vi "init.vi"(0 "Camera in":refnum<class "Camera.lvclass">, 1 "interface":u8(ring)=255 items=["FireWire"=1, "GenICam"=3, "GigE"=5, "USB"=6, "CameraLinkME4"=7, "USB3"=8, "CLHS"=11, "All"=255], 3 "error in (no error)":errorcluster) -> (7 "Camera out":refnum<class "Camera.lvclass">, 10 "error out":errorcluster)   [LabVIEW 2019, in "Camera.lvclass"]
doc: "This function is similar to init.vi but with the additional option to select the interface where\ncameras should be searched for. The default is All Interfaces. In contrast to init.vi, this function\nuses the pco.sdk function PCO_OpenCameraEx.vi to search the interfaces individually.\n\nYou should use this function instead of init.vi when:\n - You want to search for cameras at a specific interface.\n - You want to create multiple Camera objects in an application where the cameras are partially connected during operation."
uses:
  Camera.lvclass
  pco.sdk/Structures/Structures.lvlib
  pco.sdk/CameraAccess/CameraAccess.lvlib
  pco.sdk/CameraDescription/CameraDescription.lvlib
  pco.sdk/GeneralCameraStatus/GeneralCameraStatus.lvlib
  pco.convert/Convert.lvlib
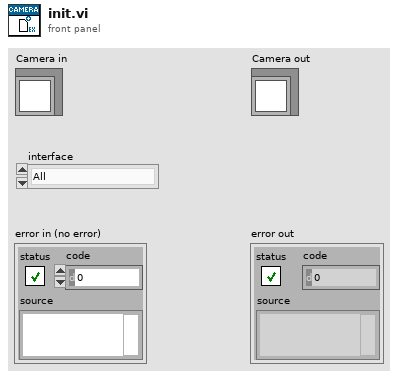
[diagram p1: front panel]
types:
  T1 = cluster{"wCamType":u16, "wCamSubType":u16, "dwSerialNumber":u32, "dwHWVersion":u32, "dwFWVersion":u32, "InterfaceType":u16, "PCO_FW_Vers":cluster{"wDeviceNum":u16, "PCO_SC2_Firmware_DESC":cluster{"szName":string, "bMinorRev":u8, "bMajorRev":u8, "wVariant":u16}[]}, "PCO_HW_Vers":cluster{"wBoardNum":u16, "PCO_SC2_Hardware_DESC":cluster{"szName":string, "wBatchNo":u16, "wRevision":u16, "wVariant":u16}[]}}
  T2 = cluster{"wSensorTypeDESC":u16, "wSensorSubTypeDESC":u16, "wMaxHorzResStdDESC":u16, "wMaxVertResStdDESC":u16, "wMaxHorzResExtDESC":u16, "wMaxVertResExtDESC":u16, "wDynResDESC":u16, "wMaxBinHorzDESC":u16, "wBinHorzSteppingDESC":u16, "wMaxBinVertDESC":u16, "wBinVertSteppingDESC":u16, "wRoiHorStepsDESC":u16, "wRoiVertStepsDESC":u16, "wNumADCsDESC":u16, "wMinSizeHorzDESC":u16, "dwPixelRateDESC":u32[], "wConvFactDESC":u16[], "sCoolingSetpoints":i16[], "wSoftRoiHorStepsDESC":u16, "wSoftRoiVertStepsDESC":u16, "wIRDESC":u16, "wMinSizeVertDESC":u16, "dwMinDelayDESC":u32, "dwMaxDelayDESC":u32, "dwMinDelayStepDESC":u32, "dwMinExposureDESC":u32, "dwMaxExposureDESC":u32, "dwMinExposureStepDESC":u32, "dwMinDelayIRDESC":u32, "dwMaxDelayIRDESC":u32, "dwMinExposureIRDESC":u32, "dwMaxExposureIRDESC":u32, "wTimeTableDESC":u16, "wDoubleImageDESC":u16, "sMinCoolSetDESC":i16, "sMaxCoolSetDESC":i16, "sDefaultCoolSetDESC":i16, "wPowerDownModeDESC":u16, "wOffsetRegulationDESC":u16, "wColorPatternDESC":u16, "wPatternTypeDESC":u16, "wNumCoolingSetpoints":u16, "dwGeneralCapsDESC1":u32, "dwGeneralCapsDESC2":u32, "dwExtSyncFrequency":u32[], "dwGeneralCapsDESC3":u32, "dwGeneralCapsDESC4":u32}
  T3 = cluster{"sharpen":bool, "adaptive_sharpen":bool, "flip_vertical":bool, "auto_minmax":bool, "min_limit":u16, "max_limit":u16, "gamma":dbl, "contrast":i32, "pco_debayer_algorithm":bool, "color_temperature":i32, "color_saturation":i32, "color_vibrance":i32, "color_tint":i32, "lut_file":path}
  T4 = cluster{"wInterfaceType":u16, "wCameraNumber":u16, "wCameraNumAtInterface":u16, "wOpenFlags":u16[], "dwOpenFlags":u32[], "wOpenPtr":u64[]}
  T5 = cluster{"iConversionFactor":i32, "iDataBits":i32, "iSensorInfoBits":i32, "iDarkOffset":i32, "strColorCoeff":dbl[], "iCamNum":i32, "hCamera":u64}
  T6 = enum16{"Undefined", "Mono8", "Mono16", "BGRA8", "RGBA8", "BGRA16", "RGBA16", "CompressedMono8"}
  T7 = map{enum16{"Undefined", "Mono8", "Mono16", "BGRA8", "RGBA8", "BGRA16", "RGBA16", "CompressedMono8"}, bool}
  T8 = map{enum16{"Undefined", "Mono8", "Mono16", "BGRA8", "RGBA8", "BGRA16", "RGBA16", "CompressedMono8"}, cluster{"sharpen":bool, "adaptive_sharpen":bool, "flip_vertical":bool, "auto_minmax":bool, "min_limit":u16, "max_limit":u16, "gamma":dbl, "contrast":i32, "pco_debayer_algorithm":bool, "color_temperature":i32, "color_saturation":i32, "color_vibrance":i32, "color_tint":i32, "lut_file":path}}
  T9 = map{enum16{"Undefined", "Mono8", "Mono16", "BGRA8", "RGBA8", "BGRA16", "RGBA16", "CompressedMono8"}, u64}
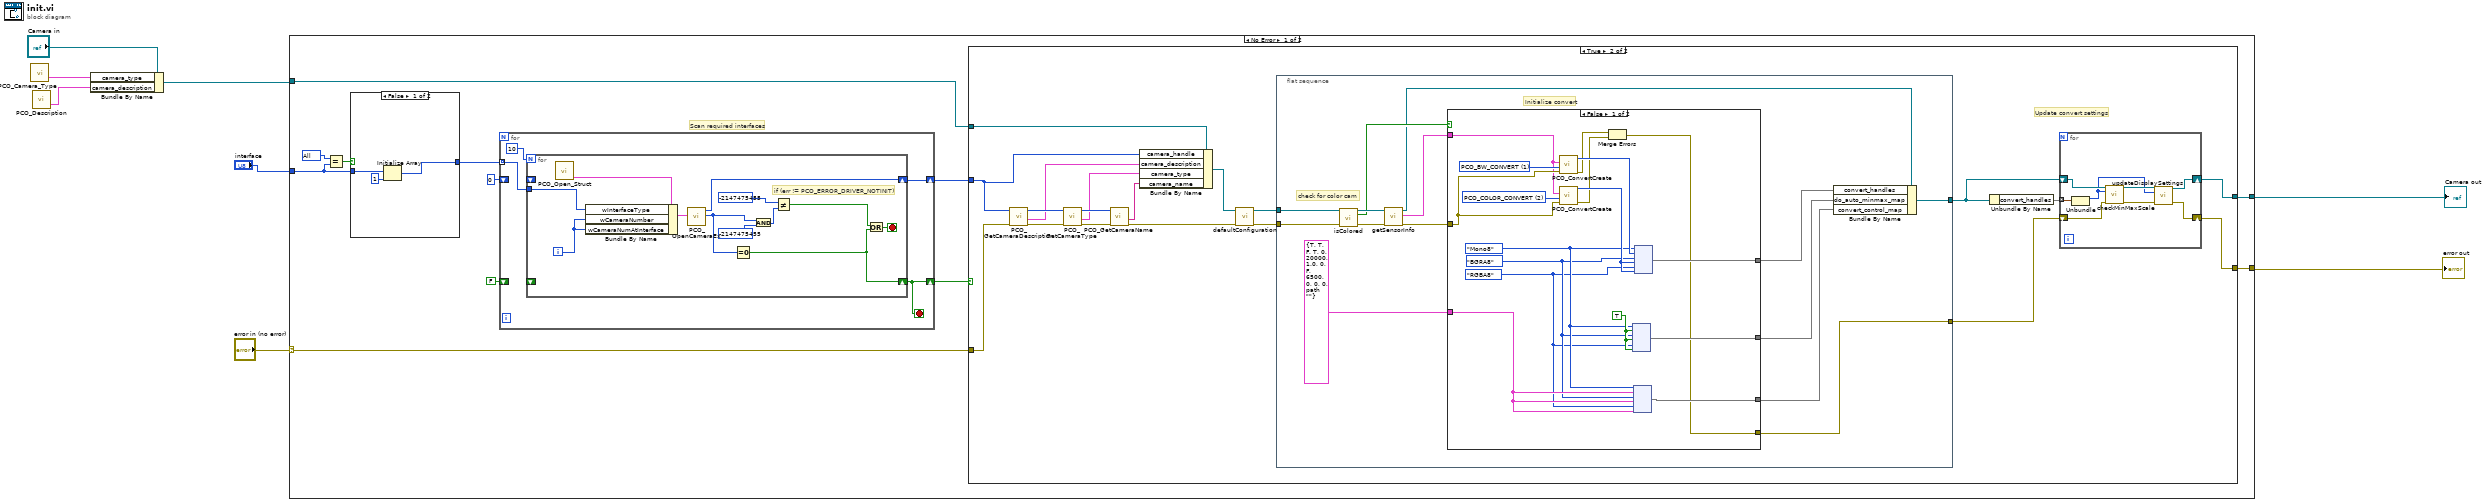
[diagram p0: block diagram]
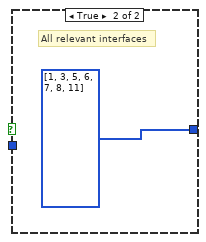
[diagram p2: hidden frame]
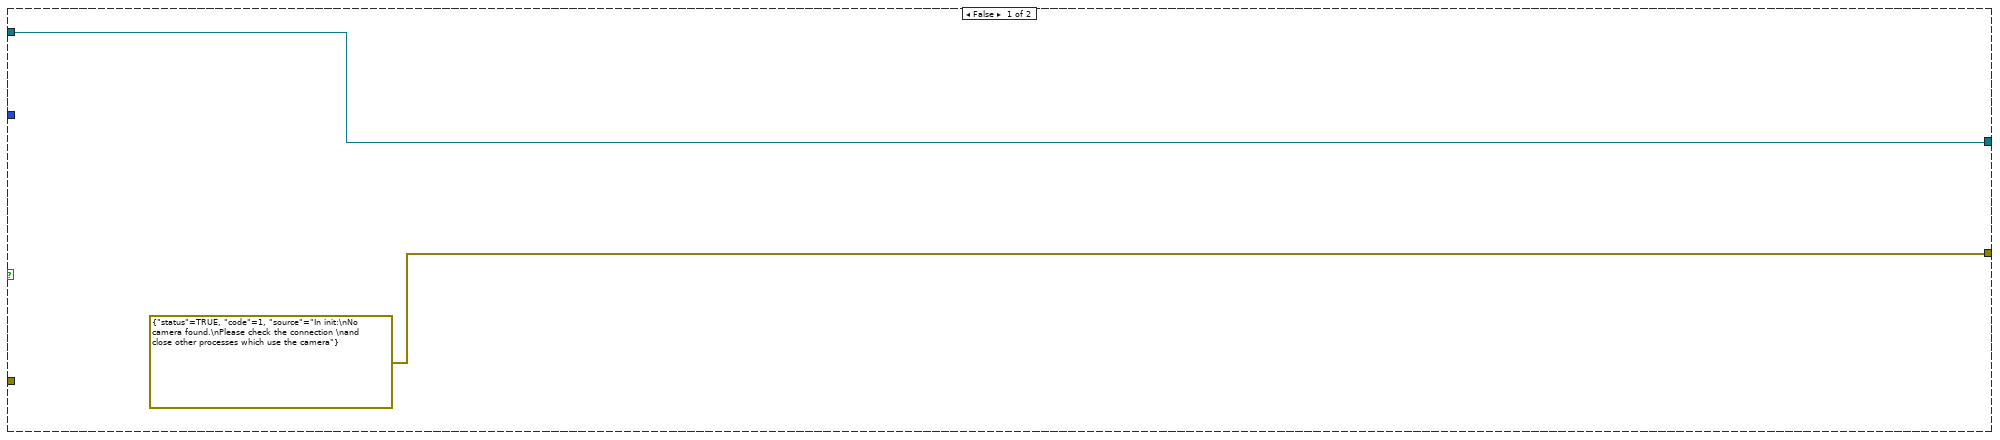
[diagram p3: hidden frame]
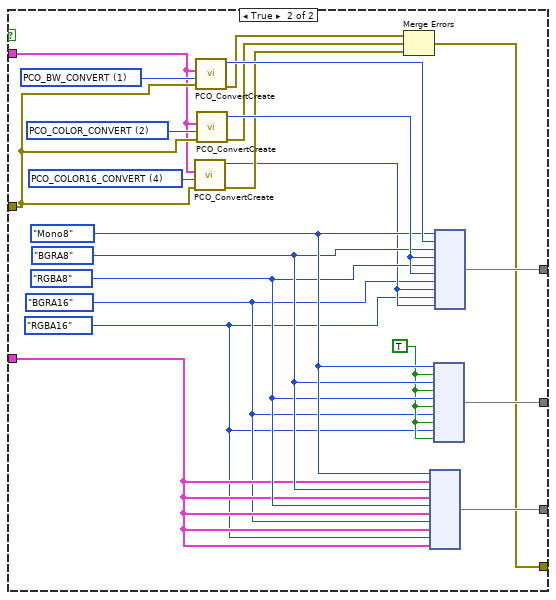
[diagram p4: hidden frame]
diagram:
  n1 = call "PCO_Camera_Type.vi"() -> ("PCO_CameraType"=w4:T1)  [unwired: 4 in, 3 out]
  n2 = call "PCO_Description.vi"() -> ("PCO_Description"=w3:T2)  [unwired: 4 in, 3 out]
  n3 = Bundle By Name(cluster="Camera in", "camera_type"=w4, "camera_description"=w3) -> (w1:refnum<class "Camera.lvclass">)
  n4 = case shown="No Error" "error in (no error)" {
    selector: "error in (no error)" -> [w9 w124]
    tunnel: [w18 w124] -> w7
    tunnel: [w16 w123] -> w6
    tunnel: w1 -> [w17 w123]
    tunnel: "interface" -> [w13 _]
    frame No Error {
      w15 = u8 255 items=["FireWire"=1, "GenICam"=3, "GigE"=5, "USB"=6, "CameraLinkME4"=7, "USB3"=8, "CLHS"=11, "All"=255] ("interface")
      # "Scan required interfaces"
      n5 = Equal?(x=w15, y=w13) -> (x = y?=w14:bool)
      n6 = case shown="False" w14 {
        tunnel: w13 -> [w39 _]
        tunnel: [w37 u8[] [1, 3, 5, 6, 7, 8, 11]] -> w10
        frame False {
          n7 = Initialize Array(w39, 1 ("dimension size")) -> (w37:u8[])
        }
        frame True {
          # "All relevant interfaces"
        }
      }
      n8 = for {
        shift-right: [w23] -> w19
        shift-left: u64 0 ("ph out") -> [_]
        shift-right: [w22] -> w20
        shift-left: FALSE -> [_]
        tunnel: w10 -> [w21] mode=indexing
        stop <- w22 stop-if-true
        n9 = for {
          N: 10 -> [_]
          tunnel: w21 -> [w35]
          shift-right: [w31] -> w22
          shift-left: _ -> [_]
          shift-right: [w29] -> w23
          shift-left: _ -> [_]
          i -> [w25]
          stop <- w30 stop-if-true
          # "if (err != PCO_ERROR_DRIVER_NOTINIT)"
          n10 = call "PCO_Open_Struct.vi"() -> ("PCO_Open_Struct"=w36:T4)  [unwired: 4 in, 4 out]
          n11 = Bundle By Name(cluster=w36, "wInterfaceType"=w35, "wCameraNumber"=w25, "wCameraNumAtInterface"=w25) -> (w34:T4)
          n12 = call "PCO_OpenCameraEx.vi"("strOpenStruct"=w34) -> ("ErrorMessage"=w26:i32, "ph out"=w29:u64)  [unwired: 8 in, 1 out]
          n13 = Equal To 0?(x=w26) -> (x = 0?=w31:bool)
          n14 = And(x=w26, y=-2147475455 ("x")) -> (x .and. y?=w28:i32)
          n15 = Not Equal?(x=-2147475455, y=w28) -> (x != y?=w32:bool)
          n16 = Or(x=w32, y=w31) -> (x .or. y?=w30:bool)
        }
      }
      n17 = case shown="True" w20 {
        tunnel: [errorcluster {"status"=TRUE, "code"=1, "source"="In init:\nNo camera found.\nPlease check the connection \nand close other processes which use the camera"} ("error out") w44] -> w18
        tunnel: w19 -> [_ w54]
        tunnel: w17 -> [w41 w60]
        tunnel: [w41 w45] -> w16
        tunnel: w9 -> [_ w61]
        frame False {
        }
        frame True {
          # "Update convert settings"
          n18 = call "PCO_GetCameraDescription.vi"("error in (no error)"=w61, "ph"=w54) -> ("error out"=w59:errorcluster, "strDescription"=w55:T2, "ph out"=w58:u64)  [unwired: 6 in, 1 out]
          n19 = call "PCO_GetCameraType.vi"("error in (no error)"=w59, "ph"=w58) -> ("error out"=w56:errorcluster, "strCamType"=w53:T1, "ph out"=w57:u64)  [unwired: 6 in, 1 out]
          n20 = call "PCO_GetCameraName.vi"("error in (no error)"=w56, "ph"=w57) -> ("error out"=w51:errorcluster, "szCameraName"=w52:string)  [unwired: 6 in, 2 out]
          n21 = Bundle By Name(cluster=w60, "camera_handle"=w54, "camera_description"=w55, "camera_type"=w53, "camera_name"=w52) -> (w50:refnum<class "Camera.lvclass">)
          n22 = call-dynamic "defaultConfiguration.vi"("error in (no error)"=w51, "Camera in"=w50) -> ("error out"=w48:errorcluster, "Camera out"=w49:refnum<class "Camera.lvclass">)  [unwired: 8 in]
          n23 = flat-sequence {
            tunnel: w49 -> [w83]
            tunnel: w48 -> [w82]
            tunnel: [w70] -> w46
            tunnel: [w74] -> w43
            frame #0 {
              # "check for color cam"
              # "Initialize convert"
              n24 = call-dynamic "isColored.vi"("Camera in"=w83, "error in (no error)"=w82) -> ("Camera out"=w80:refnum<class "Camera.lvclass">, "colored"=w79:bool, "error out"=w81:errorcluster)  [unwired: 11 in]
              n25 = call-dynamic "getSensorInfo.vi"("error in (no error)"=w81, "Camera in"=w80) -> ("error out"=w76:errorcluster, "PCO_SensorInfo"=w77:T5, "Camera out"=w75:refnum<class "Camera.lvclass">)  [unwired: 7 in]
              n26 = case shown="False" w79 {
                tunnel: [w99 w110] -> w73
                tunnel: [w100 w103] -> w72
                tunnel: T3 {"sharpen"=TRUE, "adaptive_sharpen"=TRUE, "flip_vertical"=FALSE, "auto_minmax"=TRUE, "min_limit"=0, "max_limit"=20000, "gamma"=1.0, "contrast"=0, "pco_debayer_algorithm"=FALSE, "color_temperature"=6500, "color_saturation"=0, "color_vibrance"=0, "color_tint"=0, "lut_file"=path ""} ("convert_control") -> [w97 w109]
                tunnel: [w98 w102] -> w71
                tunnel: w77 -> [w92 w111]
                tunnel: w76 -> [w93 w112]
                tunnel: [w84 w101] -> w70
                frame False {
                  w85 = T6."RGBA8" ("data_format")
                  w86 = T6."BGRA8" ("data_format")
                  w87 = T6."Mono8" ("data_format")
                  w96 = TRUE
                  w94 = 2 items=["PCO_BW_CONVERT"=1, "PCO_COLOR_CONVERT"=2, "PCO_PSEUDO_CONVERT"=3, "PCO_COLOR16_CONVERT"=4]
                  w95 = 1 items=["PCO_BW_CONVERT"=1, "PCO_COLOR_CONVERT"=2, "PCO_PSEUDO_CONVERT"=3, "PCO_COLOR16_CONVERT"=4]
                  n27 = call "PCO_ConvertCreate.vi"("error in (no error)"=w93, "iConvertType"=w95, "strSensor"=w92) -> ("error out"=w89:errorcluster, "ph out"=w91:u64)  [unwired: 6 in, 1 out]
                  n28 = call "PCO_ConvertCreate.vi"("error in (no error)"=w93, "iConvertType"=w94, "strSensor"=w92) -> ("error out"=w88:errorcluster, "ph out"=w90:u64)  [unwired: 6 in, 1 out]
                  n29 = Merge Errors(w89, w88) -> (w84:errorcluster)
                  n30 = node(w87, w96, w86, w96, w85, w96) -> (w100:T7)
                  n31 = node(w87, w97, w86, w97, w85, w97) -> (w98:T8)
                  n32 = node(w87, w91, w86, w90, w85, w90) -> (w99:T9)
                }
                frame True {
                  w104 = T6."RGBA16" ("data_format")
                  w105 = T6."BGRA16" ("data_format")
                  w113 = 4 items=["PCO_BW_CONVERT"=1, "PCO_COLOR_CONVERT"=2, "PCO_PSEUDO_CONVERT"=3, "PCO_COLOR16_CONVERT"=4]
                  w114 = T6."RGBA8" ("data_format")
                  w115 = T6."BGRA8" ("data_format")
                  w116 = T6."Mono8" ("data_format")
                  w108 = TRUE
                  w121 = 2 items=["PCO_BW_CONVERT"=1, "PCO_COLOR_CONVERT"=2, "PCO_PSEUDO_CONVERT"=3, "PCO_COLOR16_CONVERT"=4]
                  w122 = 1 items=["PCO_BW_CONVERT"=1, "PCO_COLOR_CONVERT"=2, "PCO_PSEUDO_CONVERT"=3, "PCO_COLOR16_CONVERT"=4]
                  n33 = call "PCO_ConvertCreate.vi"("error in (no error)"=w112, "iConvertType"=w113, "strSensor"=w111) -> ("error out"=w107:errorcluster, "ph out"=w106:u64)  [unwired: 6 in, 1 out]
                  n34 = call "PCO_ConvertCreate.vi"("error in (no error)"=w112, "iConvertType"=w122, "strSensor"=w111) -> ("error out"=w118:errorcluster, "ph out"=w120:u64)  [unwired: 6 in, 1 out]
                  n35 = call "PCO_ConvertCreate.vi"("error in (no error)"=w112, "iConvertType"=w121, "strSensor"=w111) -> ("error out"=w117:errorcluster, "ph out"=w119:u64)  [unwired: 6 in, 1 out]
                  n36 = Merge Errors(w118, w117, w107) -> (w101:errorcluster)
                  n37 = node(w116, w109, w115, w109, w114, w109, w105, w109, w104, w109) -> (w102:T8)
                  n38 = node(w116, w108, w115, w108, w114, w108, w105, w108, w104, w108) -> (w103:T7)
                  n39 = node(w116, w120, w115, w119, w114, w119, w105, w106, w104, w106) -> (w110:T9)
                }
              }
              n40 = Bundle By Name(cluster=w75, "convert_handles"=w73, "do_auto_minmax_map"=w72, "convert_control_map"=w71) -> (w74:refnum<class "Camera.lvclass">)
            }
          }
          n41 = Unbundle By Name(w43) -> ("convert_handles"=w47:T9)
          n42 = for {
            tunnel: w47 -> [w69] mode=indexing
            shift-right: [w68] -> w45
            shift-left: w43 -> [w66]
            shift-right: [w67] -> w44
            shift-left: w46 -> [w64]
            n43 = Unbundle(w69) -> (w62:T6)  [unwired: 1 out]
            n44 = call-dynamic "checkMinMaxScale.vi"("Camera in"=w66, "data_format"=w62, "error in (no error)"=w64) -> ("Camera out"=w65:refnum<class "Camera.lvclass">, "error out"=w63:errorcluster)  [unwired: 10 in, 1 out]
            n45 = call-dynamic "updateDisplaySettings.vi"("Camera in"=w65, "data_format"=w62, "error in (no error)"=w63) -> ("Camera out"=w68:refnum<class "Camera.lvclass">, "error out"=w67:errorcluster)  [unwired: 11 in]
          }
        }
      }
    }
    frame Error {
    }
  }
  "error out" <- w7
  "Camera out" <- w6
